vi "bmp_2_400.vi"() -> ()   [LabVIEW 2015]
panel:
  out "new 2":u32[][](array[numeric])
  out "new":u32[][](array[numeric])
  out "Array":i32[][](array[numeric])
  in  "Path 2":path
  in  "Path":path
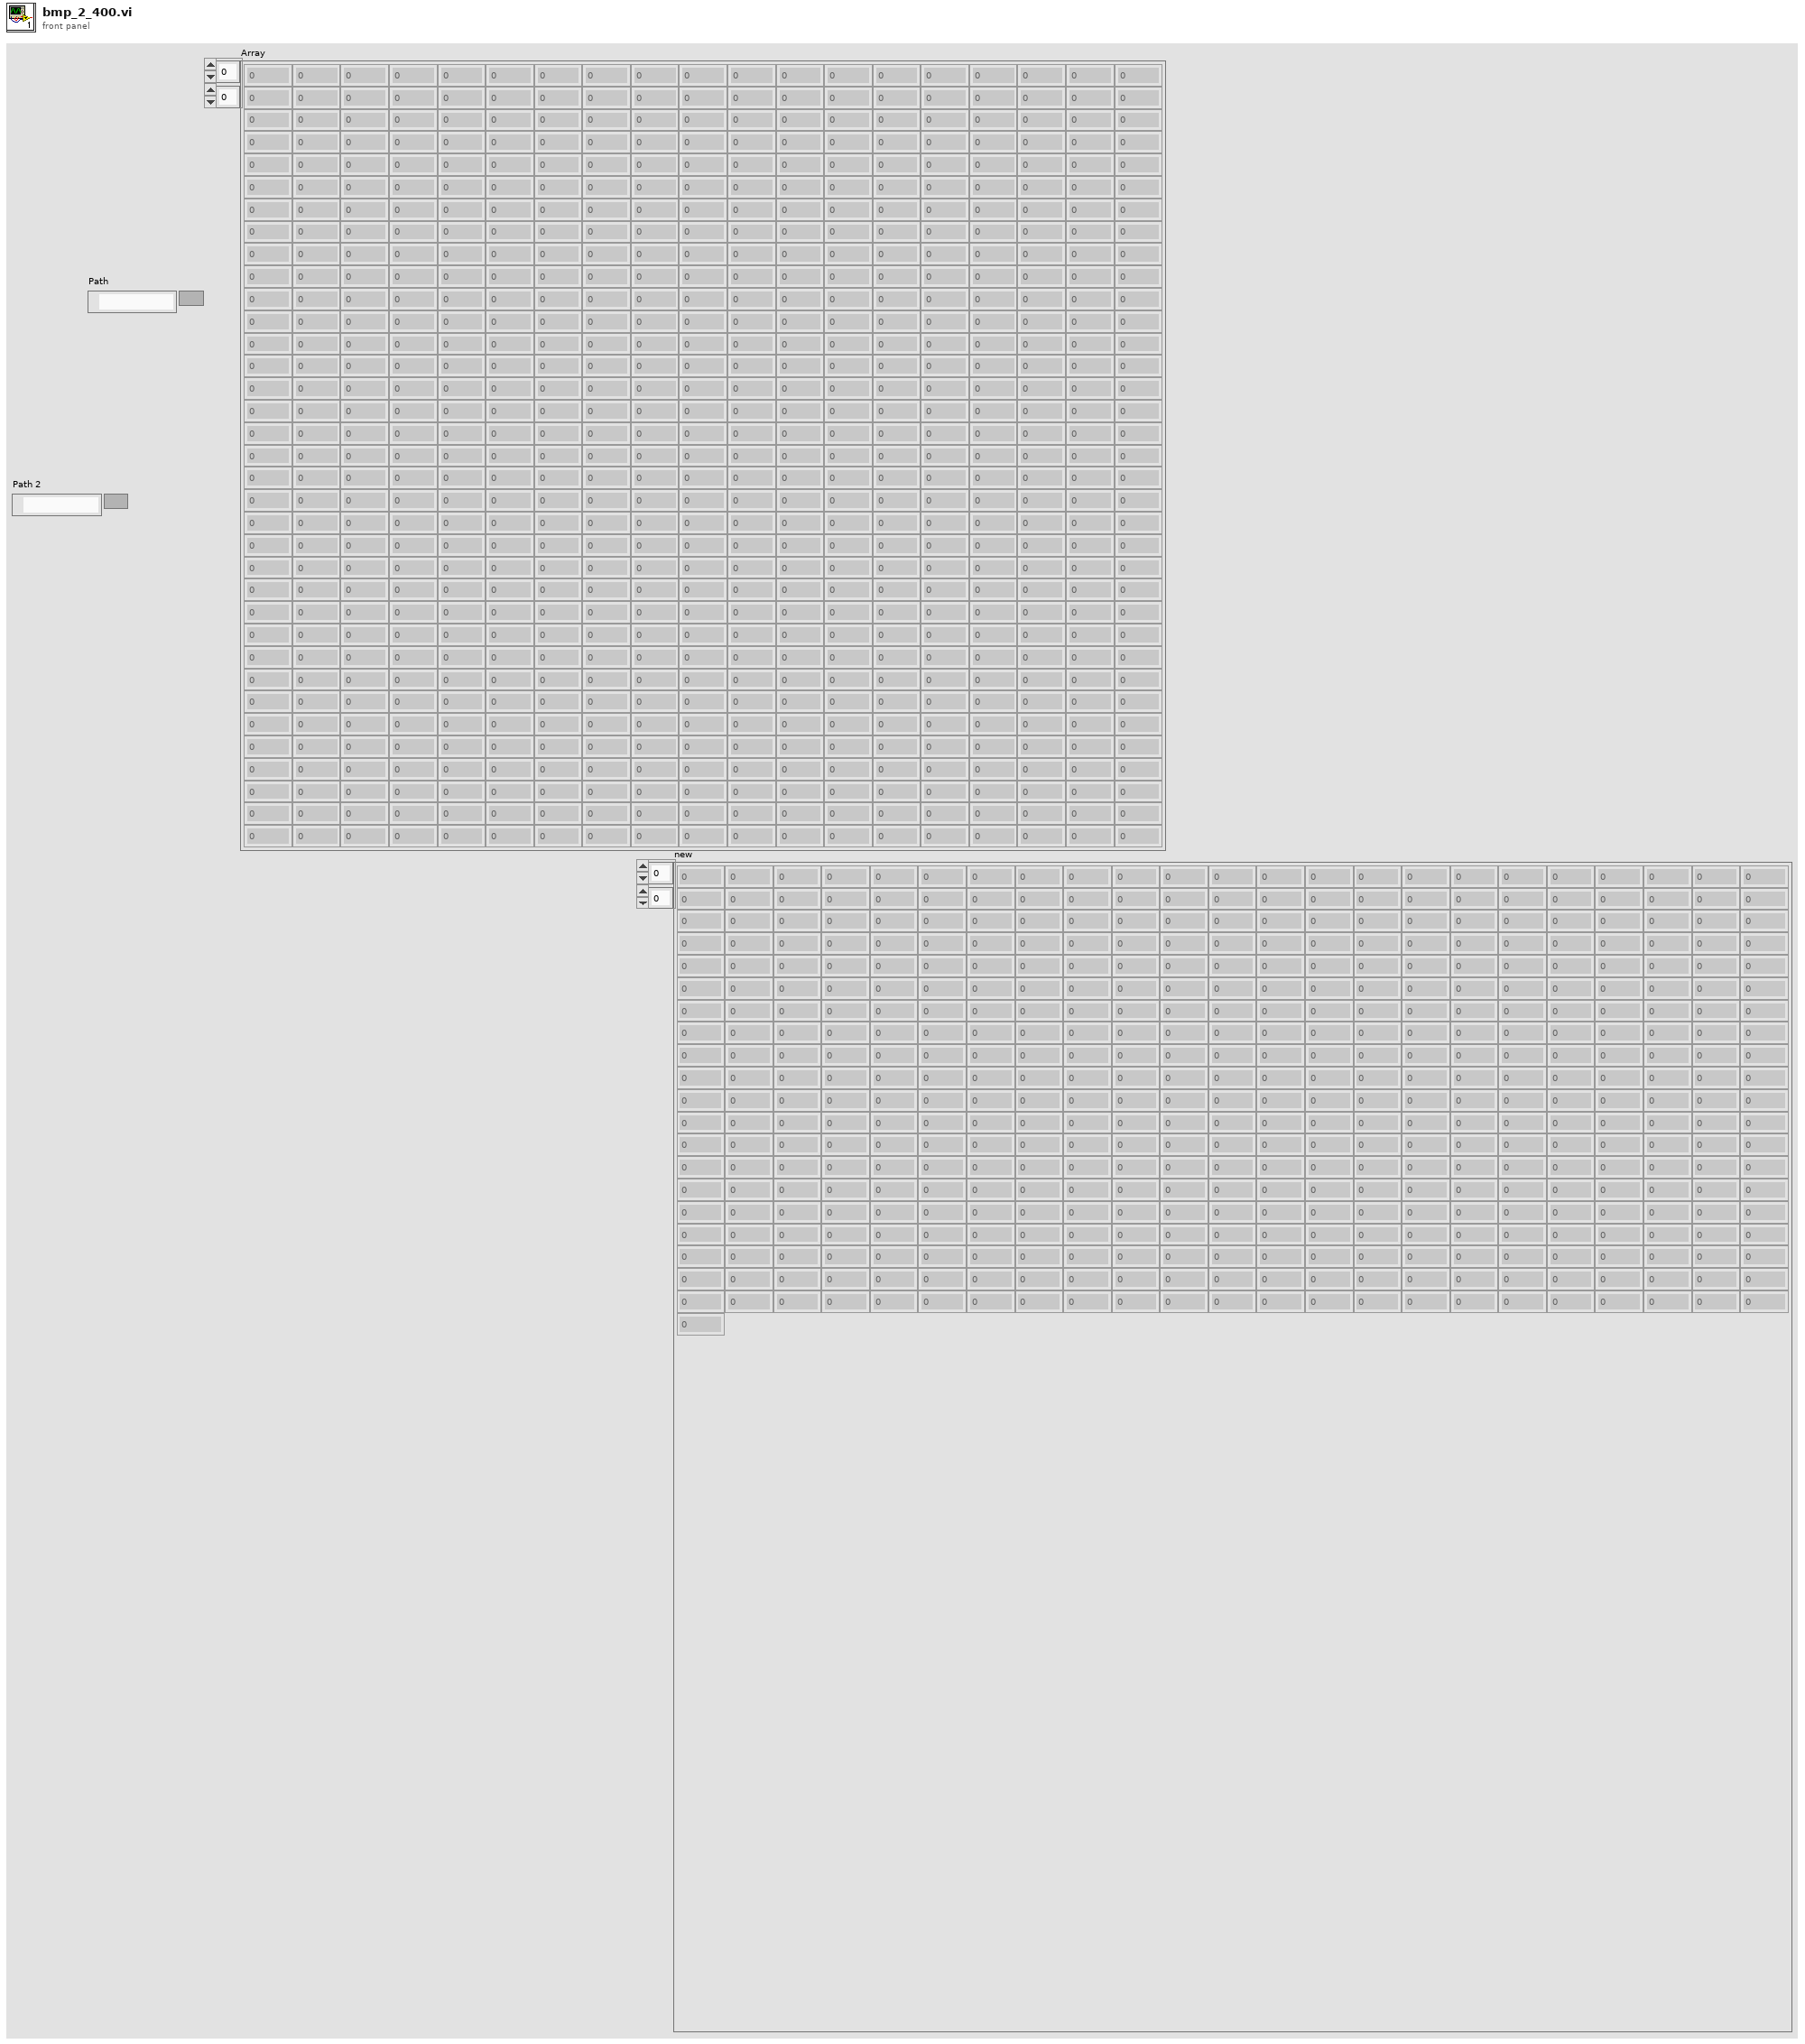
[diagram p1: front panel]
types:
  T1 = typedef "imagedata.ctl" = cluster{"image type":i32, "image depth":i32, "image":u8[], "mask":u8[], "colors":u32[], "Rectangle":cluster{"left":i16, "top":i16, "right":i16, "bottom":i16}}
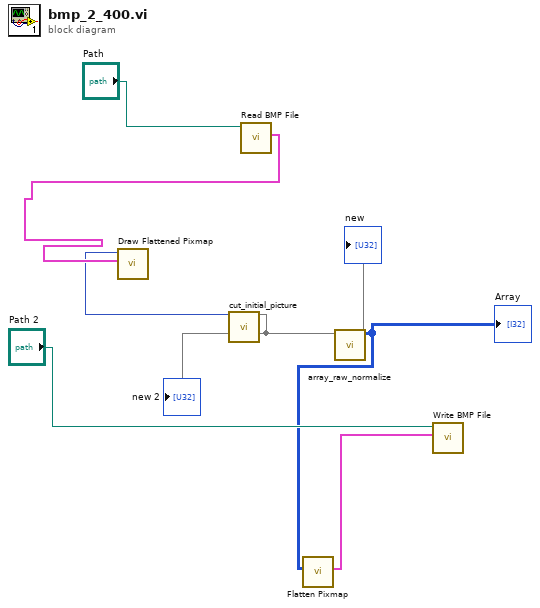
[diagram p0: block diagram]
diagram:
  n1 = call <vilib>:"Read BMP File.vi"("path to BMP file"="Path") -> ("image data"=w6:T1)  [unwired: 8 in, 2 out]
  n2 = call <vilib>:"Draw Flattened Pixmap.vi"("image data"=w6) -> ("new picture"=w5:picture)  [unwired: 8 in]
  n3 = call "cut_initial_picture.vi"("picture"=w5) -> (4:w4)  [unwired: 14 in]
  "new" <- w4
  "new 2" <- w4
  n4 = call "array_raw_normalize.vi"("array"=w4) -> ("Array"=w2:u8[][])  [unwired: 10 in]
  "Array" <- w2
  n5 = call <vilib>:"Flatten Pixmap.vi"("8-bit pixmap"=w2) -> ("image data"=w1:T1)  [unwired: 10 in]
  n6 = call <vilib>:"Write BMP File.vi"("image data"=w1, "path to BMP file"="Path 2") -> ()  [unwired: 8 in, 2 out]
